vi "RemoveEchoSerial.vi"(11 "String in":string) -> (3 "String out":string)   [LabVIEW 2017]
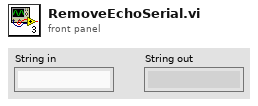
[diagram p1: front panel]
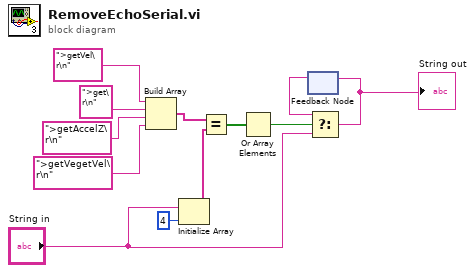
[diagram p0: block diagram]
diagram:
  n1 = Build Array(">getVel\r\n" ("x"), ">get\r\n" ("x"), ">getAccelZ\r\n" ("x"), ">getVegetVel\r\n" ("x")) -> (w2:string[])
  n2 = Initialize Array("String in", 4 ("dimension size")) -> (w1:string[])
  n3 = Equal?(x=w2, y=w1) -> (x = y?=w3:bool[])
  n4 = Or Array Elements(Boolean array=w3) -> (logical OR=w12:bool)
  n5 = feedback #1() -> (w10:string)  [unwired: 1 in]
  n6 = Select(t=w10, s=w12, f="String in") -> (s? t:f=w11:string)
  "String out" <- w11
  n7 = feedback-in #1(w11) -> ()
